vi "ForecastSummerWinter.vi"(8 "Fehler (Eingang, kein Fehler)":errorcluster, 10 "DataFlowIN (Eingang)":T1, 11 "TableName":string) -> (0 "Fehler (Ausgang)":errorcluster, 1 "Zone 2":bool, 2 "Zone 1":bool, 3 "DataFlowIN (Ausgang)":T1, 4 "Zone 3":bool, 5 "Daytime":i32, 6 "Bin-No.":u32, 7 "Night(22-6)?":bool)   [LabVIEW 2017]
uses:
  classes/DataCollector.lvclass
  classes/DataHandler.lvclass
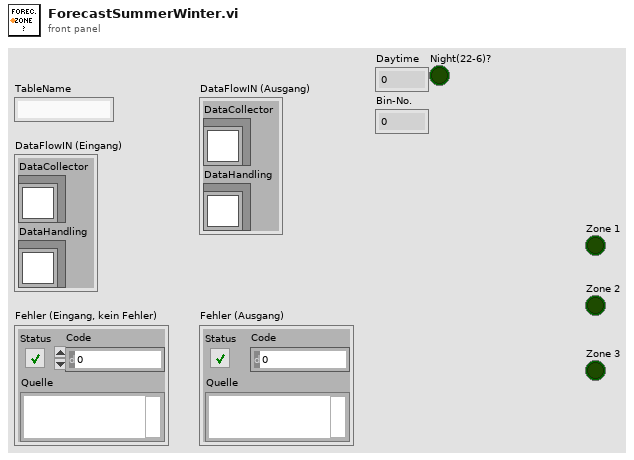
[diagram p1: front panel]
types:
  T1 = cluster{"DataCollector":refnum<class "DataCollector.lvclass">, "DataHandling":refnum<class "DataHandler.lvclass">}
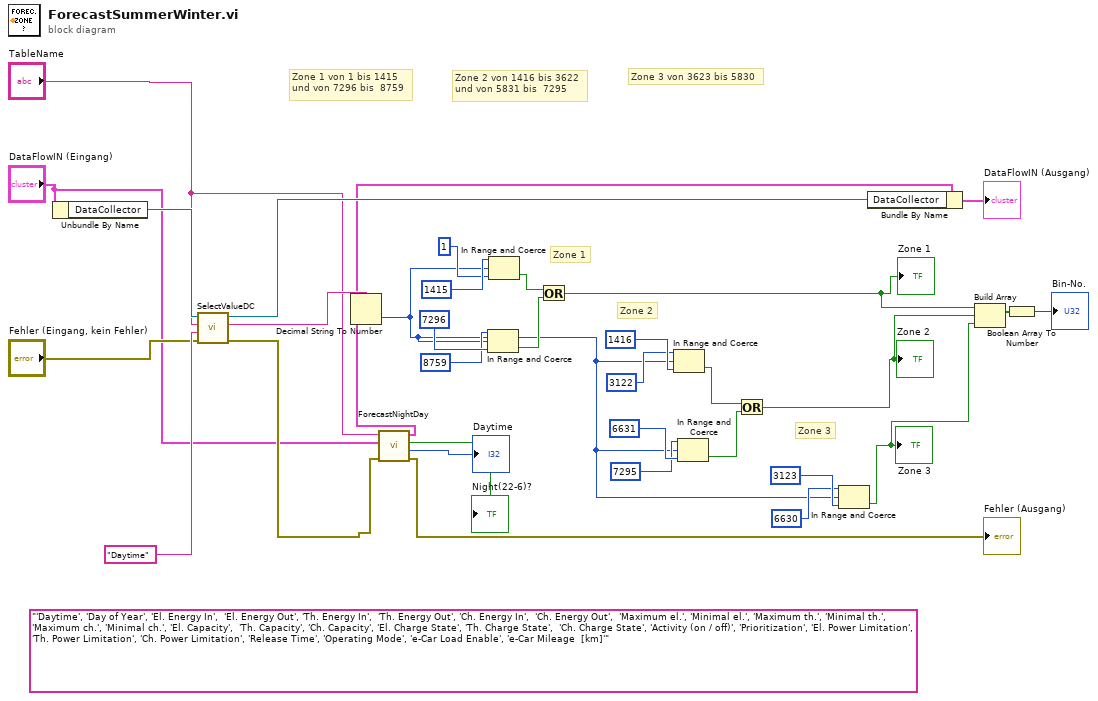
[diagram p0: block diagram]
diagram:
  (unwired) "'Daytime', 'Day of Year', 'El. Energy In',  'El. Energy Out', 'Th. Energy In',  'Th. Energy Out', 'Ch. Energy In',  'Ch. Energy Out',  'Maximum el.', 'Minimal el.', 'Maximum th.', 'Minimal th.',  'Maximum ch.', 'Minimal ch.', 'El. Capacity',  'Th. Capacity', 'Ch. Capacity', 'El. Charge State', 'Th. Charge State',  'Ch. Charge State', 'Activity (on / off)', 'Prioritization', 'El. Power Limitation',  'Th. Power Limitation', 'Ch. Power Limitation', 'Release Time', 'Operating Mode', 'e-Car Load Enable', 'e-Car Mileage  [km]'" ("string")
  # "Zone 3"
  # "Zone 2"
  # "Zone 1"
  # "Zone 3 von 3623 bis 5830"
  # "Zone 2 von 1416 bis 3622\nund von 5831 bis  7295"
  # "Zone 1 von 1 bis 1415\nund von 7296 bis  8759"
  n1 = Unbundle By Name("DataFlowIN (Eingang)") -> ("DataCollector"=w29:refnum<class "DataCollector.lvclass">)
  n2 = call-dynamic "SelectValueDC.vi"("error in (no error)"="Fehler (Eingang, kein Fehler)", "Table Row Name"="Daytime", "Unique Object Identifier"="TableName", "DataCollector in"=w29) -> ("error out"=w23:errorcluster, "Value"=w24:string, "DataCollector out"=w33:refnum<class "DataCollector.lvclass">)  [unwired: 5 in]
  n3 = Decimal String To Number(string=w24) -> (number=w1:i32)  [unwired: 2 in, 1 out]
  n4 = call "ForecastNightDay.vi"("Fehler (Eingang, kein Fehler)"=w23, "DataFlowIN (Eingang)"="DataFlowIN (Eingang)", "TableName"="TableName") -> ("Fehler (Ausgang)"=→"Fehler (Ausgang)":errorcluster, "Daytime"=→"Daytime":i32, "Night(22-6)?"=→"Night(22-6)?":bool, "DataFlowIN (Ausgang)"=w21:T1)  [unwired: 5 in]
  n5 = In Range and Coerce(upper limit=8759 ("Obergrenze"), x=w1, lower limit=7296 ("Obergrenze")) -> (In Range?=w27:bool)  [unwired: 1 out]
  n6 = In Range and Coerce(upper limit=1415 ("Obergrenze"), x=w1, lower limit=1 ("Obergrenze")) -> (In Range?=w28:bool)  [unwired: 1 out]
  n7 = Or(x=w28, y=w27) -> (x .or. y?=w18:bool)
  "Zone 1" <- w18
  n8 = In Range and Coerce(upper limit=3122 ("Obergrenze"), x=w1, lower limit=1416 ("Obergrenze")) -> (In Range?=w26:bool)  [unwired: 1 out]
  n9 = In Range and Coerce(upper limit=7295 ("Obergrenze"), x=w1, lower limit=6631 ("Obergrenze")) -> (In Range?=w25:bool)  [unwired: 1 out]
  n10 = Or(x=w26, y=w25) -> (x .or. y?=w17:bool)
  "Zone 2" <- w17
  n11 = In Range and Coerce(upper limit=6630 ("Obergrenze"), x=w1, lower limit=3123 ("Obergrenze")) -> (In Range?=w16:bool)  [unwired: 1 out]
  "Zone 3" <- w16
  n12 = Bundle By Name(cluster=w21, "DataCollector"=w33) -> (→"DataFlowIN (Ausgang)":T1)
  n13 = Build Array(w18, w17, w16) -> (w15:bool[])
  n14 = Boolean Array To Number(Boolean array=w15) -> (number=→"Bin-No.":u32)
